vi "Local to Global.vi"(9 "thetaIN":dbl, 10 "yIN":dbl, 11 "xIN":dbl) -> (2 "yOUT":dbl, 3 "xOUT":dbl)   [LabVIEW 2017]
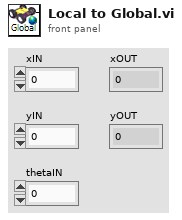
[diagram p1: front panel]
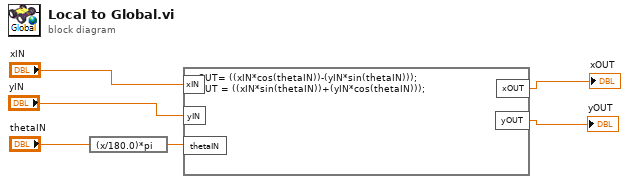
[diagram p0: block diagram]
diagram:
  n1 = expression code="(x/180.0)*pi" ("degrees to radians")("thetaIN") -> (w1:dbl)
  n2 = formula code="xOUT= ((xIN*cos(thetaIN))-(yIN*sin(thetaIN)));\nyOUT = ((xIN*sin(thetaIN))+(yIN*cos(thetaIN)));"("xIN"="xIN", "yIN"="yIN", "thetaIN"=w1) -> ("xOUT"=→"xOUT":dbl, "yOUT"=→"yOUT":dbl)
